vi "Message-handler.vi"(8 "error in (no error)":errorcluster, 10 "UI ref. in":refnum<data-value>, 11 "Data ref. in":refnum<data-value>) -> (0 "error out":errorcluster, 2 "UI ref.":refnum<data-value>, 3 "Data ref.":refnum<data-value>)   [LabVIEW 2013, in "CameraVision.lvlib" / "CV-Main.lvclass"]
doc: "Simple example of a continuous communication monitor loop.\nThe function continuously monitors the incomming (client) communication channel. At regular intervals, or after receiving a message, the client activity is reaffirmed through a 'heartbeat' message to the server.\nA new message is handled through the 'Process-received-message' function, which checks the message origins, determines the appropriate client action and executes this action."
uses:
  CV-Main.lvclass
  UI/CV-UI.lvclass
  CV-Main.lvclass/CV-Main.ctl
  Read Client.vi
  Client/Sources/CV-Client.lvclass
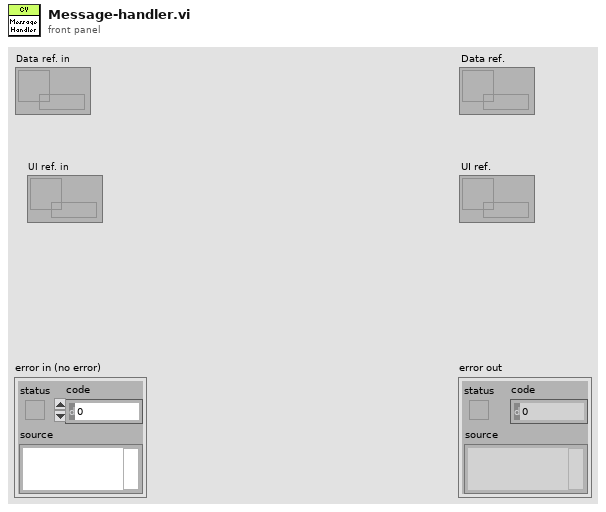
[diagram p1: front panel]
types:
  T1 = typedef "CameraVision.lvlib/CV-Client.lvclass/Object-reference.ctl" = refnum<data-value>
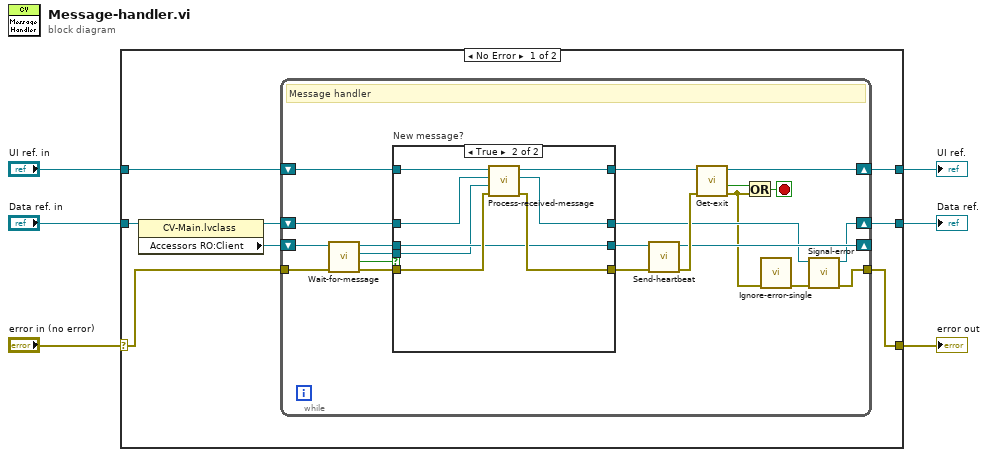
[diagram p0: block diagram]
diagram:
  n1 = case shown="No Error" "error in (no error)" {
    selector: "error in (no error)" -> [w13 w50]
    tunnel: [w12 w50] -> w5
    tunnel: "Data ref. in" -> [w14 w49]
    tunnel: [w9 w49] -> w3
    tunnel: "UI ref. in" -> [w8 w48]
    tunnel: [w7 w48] -> w1
    frame No Error {
      n2 = property class="CV-Main.lvclass"(reference=w14) -> (reference out=w10:refnum<data-value>, "Accessors RO:Client"=w11:T1)  [unwired: 1 in, 1 out]
      n3 = while {
        shift-right: [w22] -> _
        shift-left: w11 -> [w35]
        shift-right: [w18] -> w9
        shift-left: w10 -> [w26]
        tunnel: w13 -> [w33]
        tunnel: [w16] -> w12
        shift-right: [w24] -> w7
        shift-left: w8 -> [w25]
        stop <- w20 stop-if-true
        # "Message handler"
        n4 = call "Wait-for-message.vi"("error in (no error)"=w33, "Client in"=w35) -> ("error out"=w32:errorcluster, "New message?"=w30:bool, "Message"=w31:refnum<class "Message.lvclass">, "Client out"=w34:T1)  [unwired: 6 in]
        n5 = case "New message?" shown="True" w30 {
          tunnel: w34 -> [w39 w45]
          tunnel: [w39 w45] -> w29
          tunnel: w32 -> [w38 w47]
          tunnel: w31 -> [_ w44]
          tunnel: [w38 w46] -> w28
          tunnel: w26 -> [w37 w43]
          tunnel: [w37 w42] -> w19
          tunnel: w25 -> [w36 w41]
          tunnel: [w36 w40] -> w23
          frame False {
          }
          frame True {
            n6 = call "Process-received-message.vi"("error in (no error)"=w47, "Message"=w44, "Data ref. in"=w43, "UI ref. in"=w41) -> ("error out"=w46:errorcluster, "Data ref."=w42:refnum<data-value>, "UI ref."=w40:refnum<data-value>)  [unwired: 5 in]
          }
        }
        n7 = call "Send-heartbeat.vi"("error in (no error)"=w28, "Client in"=w29) -> ("error out"=w27:errorcluster, "Client out"=w22:T1)  [unwired: 8 in]
        n8 = call "Get-exit.vi"("error in (no error)"=w27, "UI ref. in"=w23) -> ("error out"=w17:errorcluster, "Exit?"=w21:bool, "UI ref."=w24:refnum<data-value>)  [unwired: 7 in]
        n9 = Or(x=w21, y=w17) -> (x .or. y?=w20:bool)
        n10 = call "Ignore-error-single.vi"("error in (no error)"=w17) -> ("error out"=w15:errorcluster)  [unwired: 10 in]
        n11 = call "Signal-error.vi"("error in (no error)"=w15, "Data ref. in"=w19) -> ("error out"=w16:errorcluster, "Data ref."=w18:refnum<data-value>)  [unwired: 8 in]
      }
    }
    frame Error {
    }
  }
  "error out" <- w5
  "Data ref." <- w3
  "UI ref." <- w1
